vi "Configure from DBC.vi"(8 "error in":errorcluster, 11 "PCAN in":refnum<class "PCAN.lvclass">) -> (0 "error out":errorcluster, 3 "PCAN out":refnum<class "PCAN.lvclass">)   [LabVIEW 2023, in "PCAN.lvclass"]
uses:
  PCAN.lvclass
  D:/git/HAL/HAL GOOP4/Configuration/Configuration JSON/Configuration JSON Base/CFG JSON.lvclass
  Configuration/Configuration JSON/Configuration JSON Base/CFG JSON.lvclass/CFG JSON.ctl
  PCAN.lvclass/PCAN.ctl
  e876bc77-3914-497d-9dbf-46d43ff41845.vi
  e876bc77-3914-497d-9dbf-46d43ff41845.vi/a4169a97-72fc-4003-a778-603cf20cafa0.vi
  <vilib>/JDP Science/JSONtext/Find Item.vi
  <vilib>/JDP Science/JSONtext/Next JSON Value.vi
  <vilib>/JDP Science/JSONtext/String Subset.vi
  <vilib>/JDP Science/JSONtext/Parsing/Advance past next JSON Value (inlined COPY).vi
  <vilib>/JDP Science/JSONtext/Parsing/Advance past whitespace.vi
  <vilib>/JDP Science/JSONtext/Parsing/Advance past String.vi
  <vilib>/JDP Science/JSONtext/Parsing/Advance past Number.vi
  <vilib>/JDP Science/JSONtext/Parsing/Advance past Line Ending.vi
  <vilib>/JDP Science/JSONtext/Parsing/Parse Full Path or Item Name.vi
  <vilib>/JDP Science/JSONtext/Parsing/Advance past Array.vi
  <vilib>/JDP Science/JSONtext/Parsing/Advance past Object.vi
  <vilib>/JDP Science/JSONtext/support/Error Cluster From Code.vi
  <vilib>/JDP Science/JSONtext/Offset/Find Item Locations by Path.vi
  <vilib>/JDP Science/JSONtext/JSON text to Variant.vi
  <vilib>/Utility/error.llb/Error Cluster From Error Code.vi
  <vilib>/xnet/xnet.llb/XNET Create Session (Conversion).vi
  <vilib>/JDP Science/JSONtext/LVClass Serializer/JSONtext LVClass Serializer.lvclass
  Configuration/Configuration JSON/Configuration JSON Base/CFG JSON.lvclass
  <resource>/objmgr/xnet.rc
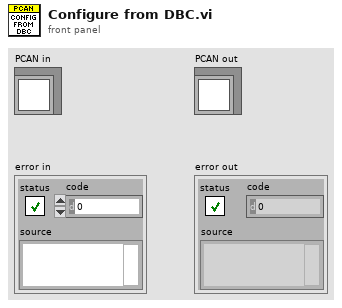
[diagram p1: front panel]
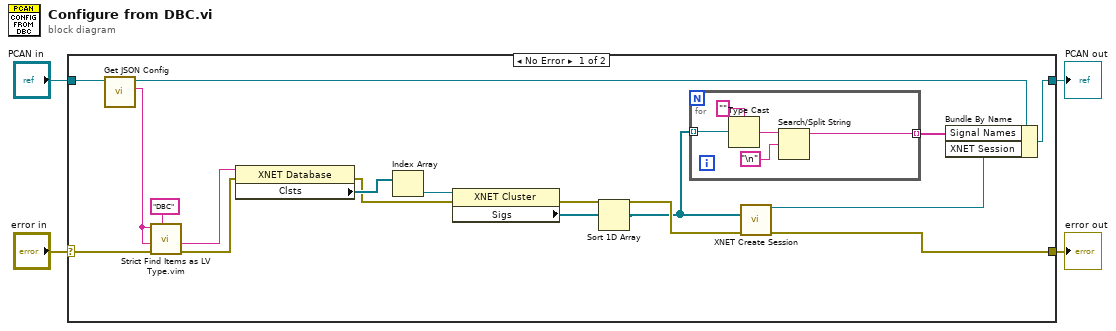
[diagram p0: block diagram]
diagram:
  n1 = case shown="No Error" "error in" {
    selector: "error in" -> [w20 w28]
    tunnel: [w7 w28] -> w3
    tunnel: [w18 w27] -> w1
    tunnel: "PCAN in" -> [w21 w27]
    frame No Error {
      n2 = call "Get JSON Config.vi"("CFG Base in"=w21) -> ("<JSON>Config>"=w16:string, "CFG Base out"=w11:refnum<class "PCAN.lvclass">)  [unwired: 9 in]
      n3 = call "Strict Find Items as LV Type.vim"("$Path or Item Name"="DBC", "error in"=w20, "Data Type and Default Value"=w16, "JSON"=w16) -> ("error out"=w14:errorcluster, "Data out"=w15:string)  [unwired: 6 in]
      n4 = property class="XNET Database"(reference=w15, error in=w14) -> (error out=w13:errorcluster, "Clsts"=w19:refnum<k21>[])  [unwired: 1 out]
      n5 = Index Array(array=w19) -> (element=w9:refnum<k21>)  [unwired: 1 in]
      n6 = property class="XNET Cluster"(reference=w9, error in=w13) -> (error out=w8:errorcluster, "Sigs"=w6:refnum<k21>[])  [unwired: 1 out]
      n7 = Sort 1D Array(array=w6) -> (sorted array=w5:refnum<k21>[])
      n8 = for {
        tunnel: w5 -> [w26] mode=indexing
        tunnel: [w23] -> w10 mode=indexing
        n9 = Type Cast(type="", x=w26) -> (*(type *) &x=w24:string)
        n10 = Search/Split String(string=w24, search string/char (-)="\n") -> (substring before match=w23:string)  [unwired: 1 in, 2 out]
      }
      n11 = call-poly <vilib>:"XNET Create Session.vi"("signal list"=w5, "error in (no error)"=w8) -> ("session out"=w12:refnum<k21>, "error out"=w7:errorcluster)  [unwired: 12 in]
      n12 = Bundle By Name(cluster=w11, "Signal Names"=w10, "XNET Session"=w12) -> (w18:refnum<class "PCAN.lvclass">)
    }
    frame Error {
    }
  }
  "error out" <- w3
  "PCAN out" <- w1
